vi "APS write d output.vi"(8 "error in (no error)":errorcluster caption="错误输入（无错误）", 9 "DO_Data":i32, 10 "DO_Group":i32, 11 "Board_ID":i32) -> (0 "error out":errorcluster caption="错误输出", 3 "function return":i32)   [LabVIEW 2017, in "APS168.lvlib"]
doc: "I32 FNTYPE APS_write_d_output(I32 Board_ID, I32 DO_Group, I32 DO_Data);"
uses:
  APS168.lvlib
  APS168.dll
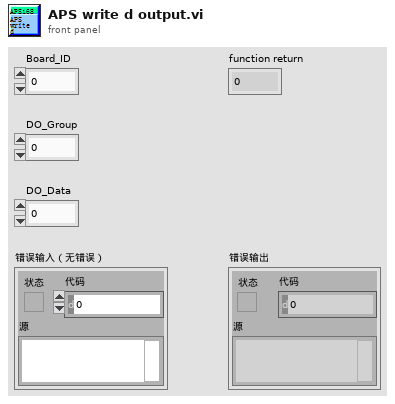
[diagram p1: front panel]
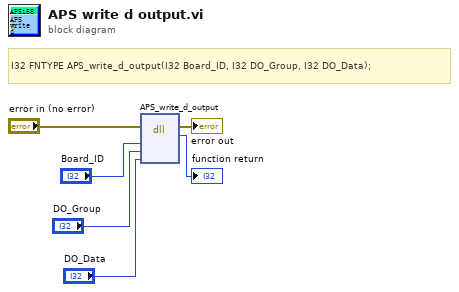
[diagram p0: block diagram]
diagram:
  # "I32 FNTYPE APS_write_d_output(I32 Board_ID, I32 DO_Group, I32 DO_Data);"
  n1 = dll-call lib="PTH2Iabs E迈治LV范例testSubVIsADLINKMotion204c\nAPS168.dll" fn="APS_write_d_output"(error in="error in (no error)", "Board_ID"="Board_ID", "DO_Group"="DO_Group", "DO_Data"="DO_Data") -> (error out=→"error out":errorcluster, "返回类型"=→"function return":i32)  [unwired: 5 in, 1 out]
